vi "Write To I16 File.vi"(4 "append to file? (new file:F)":bool caption="An Datei anhängen? (Neue Datei:F)", 5 "1D array":i16[](array[numeric]) caption="1D-Array", 6 "2D array":i16[][](array[numeric]) caption="2D-Array", 7 "file path (dialog if empty)":path caption="Dateipfad (Dialog, wenn leer)") -> (1 "new file path (Not A Path if cancelled)":path caption="Neuer Dateipfad (Kein Pfad, wenn abgebrochen)")   [LabVIEW 2009]
doc: "Schreibt ein 2D- oder 1D-Array aus vorzeichenbehafteten Integern in eine neue Bytestream-Datei oder hängt die Daten an eine vorhandene Datei an."
panel:
  in  "prompt":string="Datei zum Schreiben auswählen." caption="Eingabeaufforderung"
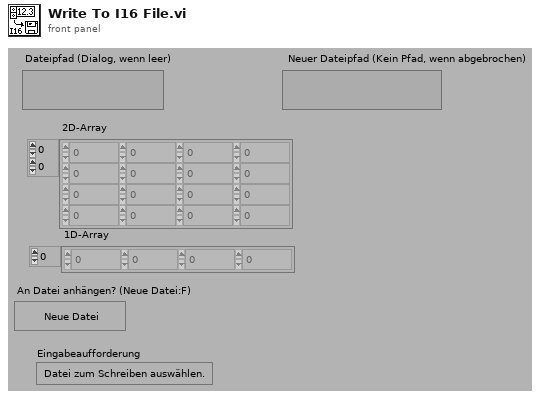
[diagram p1: front panel]
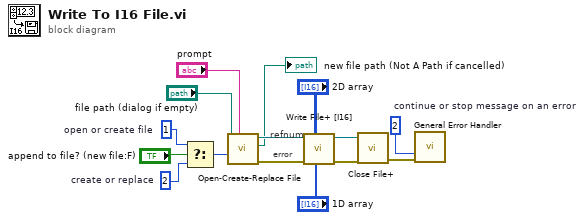
[diagram p0: block diagram]
diagram:
  w4 = i16 2  # create or replace
  w13 = 2  # continue or stop message on an error
  w8 = i16 1  # open or create file
  # "error"
  # "refnum"
  n1 = Select(t=w8, s="append to file? (new file:F)", f=w4) -> (s? t:f=w10:i16)
  n2 = call "Open-Create-Replace File.vi"("prompt"="prompt", "function (open:0)"=w10, "file path"="file path (dialog if empty)") -> ("error out"=w14:errorcluster, "new file path"=→"new file path (Not A Path if cancelled)":path, "refnum"=w3:refnum<file>)  [unwired: 5 in, 1 out]
  n3 = call "Write File+ [I16].vi"("1D array"="1D array", "2D array"="2D array", "error in (no error)"=w14, "refnum"=w3) -> ("error out"=w12:errorcluster, "dup refnum"=w11:refnum<file>)  [unwired: 5 in, 1 out]
  n4 = call "Close File+.vi"("error in (no error)"=w12, "refnum"=w11) -> ("error out"=w9:errorcluster)  [unwired: 3 in, 2 out]
  n5 = call <vilib>:"General Error Handler.vi"("type of dialog (OK msg:1)"=w13, "error in (no error)"=w9) -> ()  [unwired: 9 in, 5 out]
